vi "wait for udp trigger.vi"(8 "error in (no error)":errorcluster, 11 "Timeout":dbl=5000.0) -> (0 "No error":errorcluster)   [LabVIEW 2020]
panel:
  out "time in range?":bool
  out "shot time - current 2":dbl
  out "ms timestamp network trigger":dbl format="%#_15g"
  out "shot time - current":dbl
  out "1st read":errorcluster
  out "2nd udp error":errorcluster
  out "data out 2":string
  out "data out":string
  out "loops to clear buffer":i32
  out "current time":timestamp
  out "wait time":u32
  out "connection ID":refnum<k16>
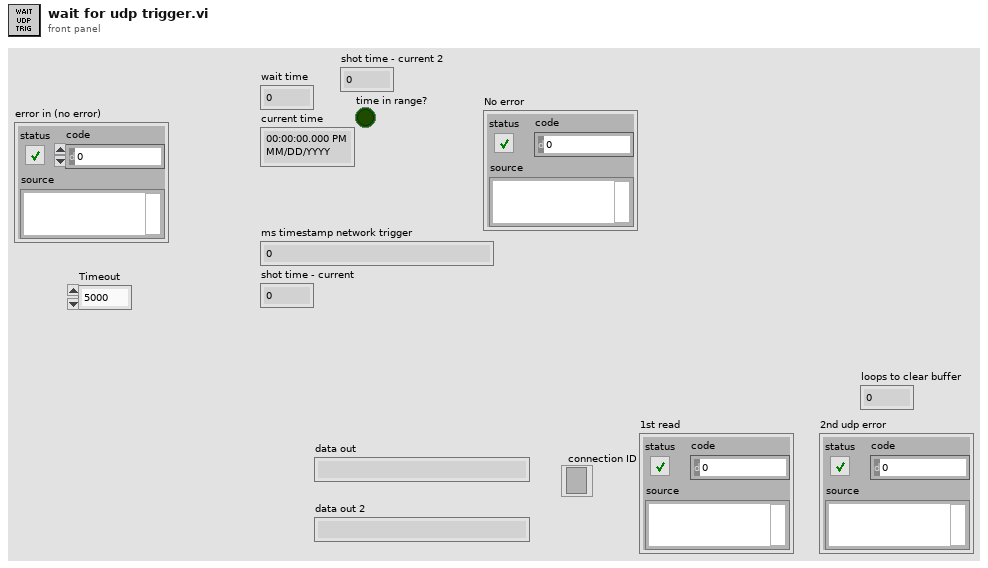
[diagram p1: front panel]
types:
  T1 = enum32{"Invalid", "Standard", "Closed", "Hidden", "Minimized", "Maximized"}
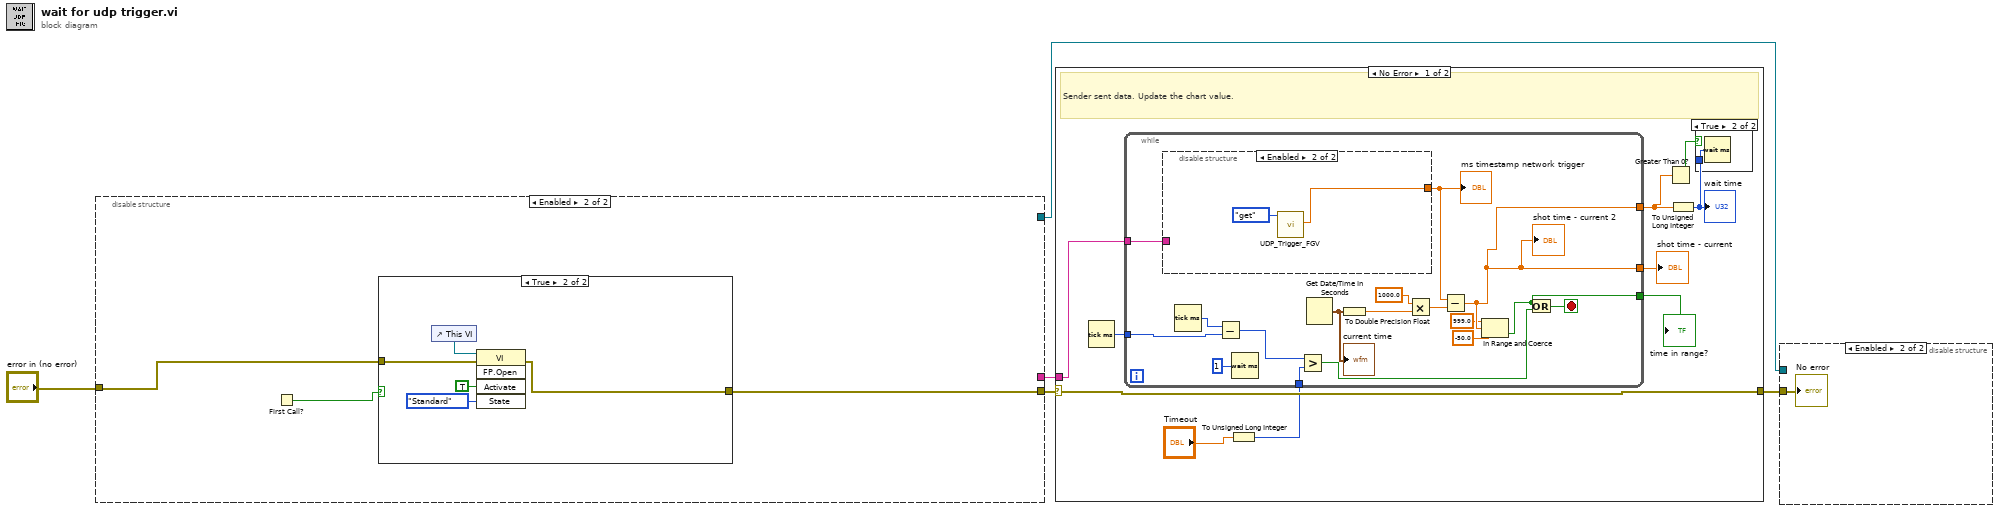
[diagram p0: block diagram]
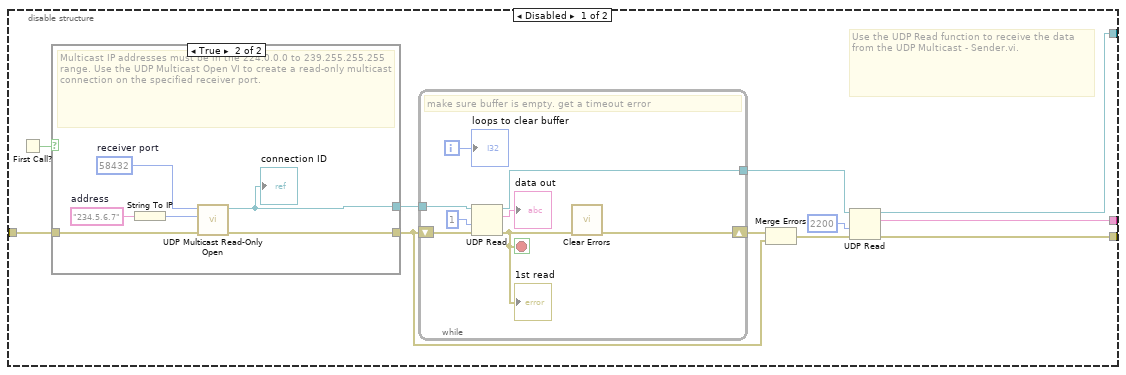
[diagram p2: hidden frame]
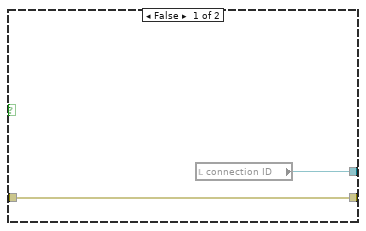
[diagram p3: hidden frame]
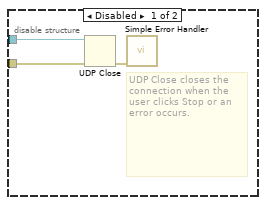
[diagram p5: hidden frame]
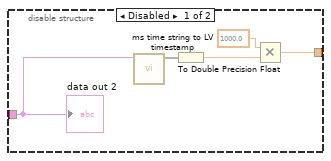
[diagram p7: hidden frame]
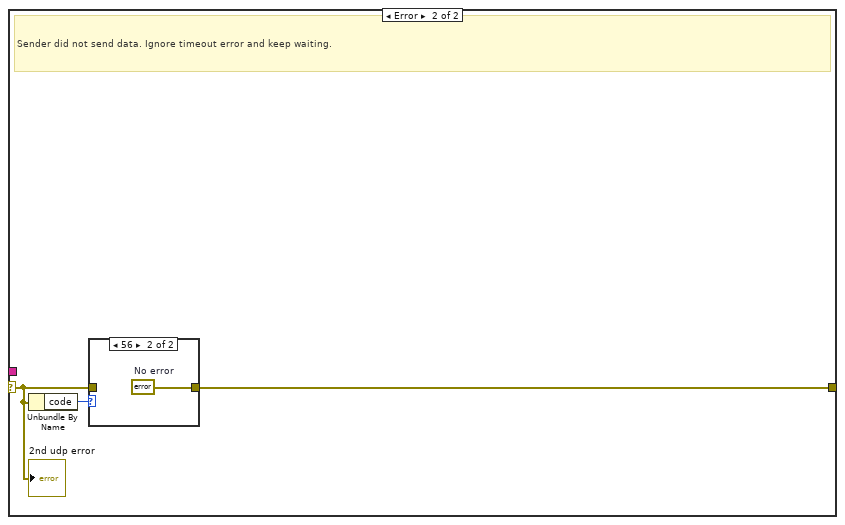
[diagram p8: hidden frame]
diagram:
  n1 = disable-structure shown="Enabled" {
    disable-tunnel: "error in (no error)" -> [w16 w34]
    disable-tunnel: [w14 w35] -> w4
    disable-tunnel: [w13 _] -> w3
    disable-tunnel: [w11 _] -> w1
    frame Disabled {
      # "Use the UDP Read function to receive the data from the UDP Multicast - Sender.vi."
      n2 = First Call?() -> (First Call?: T/F=w15:bool)
      n3 = case shown="True" w15 {
        tunnel: [w26 w31] -> w9
        tunnel: [w25 w27] -> w7
        tunnel: w16 -> [w26 w28]
        frame False {
          n4 = local read "connection ID"() -> (w25:refnum<k16>)
        }
        frame True {
          w30 = u16 58432  # receiver port
          w32 = "234.5.6.7"  # address
          # "Multicast IP addresses must be in the 224.0.0.0 to 239.255.255.255 range. Use the UDP Multicast Open VI to create a read-only multicast connection on the specified receiver port."
          n5 = String To IP(1:w32) -> (0:w29:u32)
          n6 = call "UDP Multicast Read-Only Open.vi"("error in (no error)"=w28, "multicast addr"=w29, "port"=w30) -> ("error out"=w31:errorcluster, "connection ID"=w27:refnum<k16>)  [unwired: 6 in, 1 out]
          "connection ID" <- w27
        }
      }
      n7 = while {
        shift-right: [w23] -> w10
        shift-left: w9 -> [w22]
        tunnel: w7 -> [w20]
        tunnel: [w19] -> w6
        i -> [w18]
        stop <- w21 stop-if-true
        # "make sure buffer is empty. get a timeout error"
        n8 = UDP Read(connection ID=w20, timeout ms (25000)=1, 8:w22) -> (data out=→"data out":string, error out=w21:errorcluster, 3:w19:refnum<k16>)  [unwired: 3 out]
        "1st read" <- w21
        n9 = call "Clear Errors.vi"("error in (no error)"=w21) -> ("error out"=w23:errorcluster)  [unwired: 5 in, 1 out]
        "loops to clear buffer" <- w18
      }
      n10 = Merge Errors(w10, w9) -> (w8:errorcluster)
      n11 = UDP Read(connection ID=w6, timeout ms (25000)=2200, 8:w8) -> (data out=w13:string, error out=w14:errorcluster, 3:w11:refnum<k16>)  [unwired: 3 out]
    }
    frame Enabled {
      n12 = First Call?() -> (First Call?: T/F=w33:bool)
      n13 = case shown="True" w33 {
        tunnel: [w36 w40] -> w35
        tunnel: w34 -> [w36 w39]
        frame False {
        }
        frame True {
          n14 = control-ref of="This VI"() -> (w41:refnum<vi>)
          n15 = invoke class="VI" method="FP.Open"(reference=w41, error in=w39, "Activate"=TRUE ("Activate?"), "State"=T1."Standard") -> (error out=w40:errorcluster)  [unwired: 1 in, 4 out]
        }
      }
    }
  }
  n16 = case shown="No Error" w4 {
    selector: w4 -> [w51 w78]
    tunnel: w3 -> [w50 _]
    tunnel: [w51 w77] -> w2
    frame No Error {
      # "Sender sent data. Update the chart value."
      n17 = Tick Count (ms)() -> (millisecond timer value=w48:u32)
      n18 = To Unsigned Long Integer(number="Timeout") -> (unsigned 32bit integer=w46:u32)
      n19 = while {
        tunnel: w50 -> [w69]
        tunnel: [w56] -> w45
        tunnel: w48 -> [w62]
        tunnel: w46 -> [w57]
        tunnel: [w56] -> w43
        tunnel: [w53] -> w42
        stop <- w59 stop-if-true
        n20 = disable-structure shown="Enabled" {
          disable-tunnel: w69 -> [w74 _]
          disable-tunnel: [w70 w75] -> w65
          frame Disabled {
            n21 = call "ms time string to LV timestamp.vi"("String"=w74) -> ("Time Stamp"=w71:timestamp)  [unwired: 10 in]
            n22 = To Double Precision Float(number=w71) -> (double precision float=w73:dbl)
            n23 = Multiply(x=1000.0 ("y"), y=w73) -> (x*y=w70:dbl)
            "data out 2" <- w74
          }
          frame Enabled {
            n24 = call "UDP_Trigger_FGV.vi"("command"=enum16{"set", "get", "reset"}."get") -> ("ms timestamp network trigger out"=w75:dbl)  [unwired: 10 in]
          }
        }
        "ms timestamp network trigger" <- w65
        n25 = Tick Count (ms)() -> (millisecond timer value=w63:u32)
        n26 = Subtract(x=w63, y=w62) -> (x-y=w61:u32)
        n27 = Wait (ms)(milliseconds to wait=u32 1) -> ()  [unwired: 1 out]
        n28 = Greater?(x=w61, y=w57) -> (0:w60:bool)
        n29 = Get Date/Time In Seconds() -> (seconds since 1Jan1904=w68:timestamp)
        "current time" <- w68
        n30 = To Double Precision Float(number=w68) -> (double precision float=w66:dbl)
        n31 = Multiply(x=1000.0 ("y"), y=w66) -> (x*y=w64:dbl)
        n32 = Subtract(x=w65, y=w64) -> (x-y=w56:dbl)
        "shot time - current 2" <- w56
        n33 = In Range and Coerce(upper limit=999.0, x=w56, lower limit=-50.0) -> (In Range?=w53:bool)  [unwired: 1 out]
        n34 = Or(x=w53, y=w60) -> (x .or. y?=w59:bool)
      }
      "shot time - current" <- w43
      "time in range?" <- w42
      n35 = Greater Than 0?(x=w45) -> (x > 0?=w44:bool)
      n36 = To Unsigned Long Integer(number=w45) -> (unsigned 32bit integer=w49:u32)
      "wait time" <- w49
      n37 = case shown="True" w44 {
        tunnel: w49 -> [_ w52]
        frame False {
        }
        frame True {
          n38 = Wait (ms)(milliseconds to wait=w52) -> ()  [unwired: 1 out]
        }
      }
    }
    frame Error {
      # "Sender did not send data. Ignore timeout error and keep waiting."
      n39 = Unbundle By Name(w78) -> ("code"=w79:i32)
      n40 = case shown="56" w79 {
        tunnel: w78 -> [w80 _]
        tunnel: [w80 w81] -> w77
        frame Default {
        }
        frame 56 {
          w81 = errorcluster {"status"=FALSE, "code"=0, "source"=""}  # No error
        }
      }
      "2nd udp error" <- w78
    }
  }
  n41 = disable-structure shown="Enabled" {
    disable-tunnel: w1 -> [w84 _]
    disable-tunnel: w2 -> [w82 w85]
    frame Disabled {
      # "UDP Close closes the connection when the user clicks Stop or an error occurs."
      n42 = UDP Close(connection ID=w84, 8:w82) -> (error out=w83:errorcluster)  [unwired: 1 out]
      n43 = call "Simple Error Handler.vi"("error in (no error)"=w83) -> ()  [unwired: 1 in, 8 out]
    }
    frame Enabled {
      "No error" <- w85
    }
  }
